vi "Get Formula String Dialog.vi"(8 "error in (no error)":errorcluster, 10 "Variable (x)":string="x", 11 "Formula Name (f(x))":string="f(x)") -> (0 "error out":errorcluster, 1 "Cancelled?":bool, 3 "Formula":string)   [LabVIEW 2019, in "XY Graph Add-Ons.lvlib"]
doc: "Displays a standard dialog box that prompts users to enter information, such as a user name and password.\n--------------------\n\nThis Express VI is configured as follows:\n\nMessage to Display to the User:\nThe inputs are: \nText Entry Box: Formula"
uses:
  XY Graph Add-Ons.lvlib
panel:
  in  "Formula":string caption="y' ="
  out "String":string="Enter formula using x as variable (e.g.: 3.0*x**2 - 4.32):"
  in  "Cancel":bool
  in  "OK":bool caption="OK2"
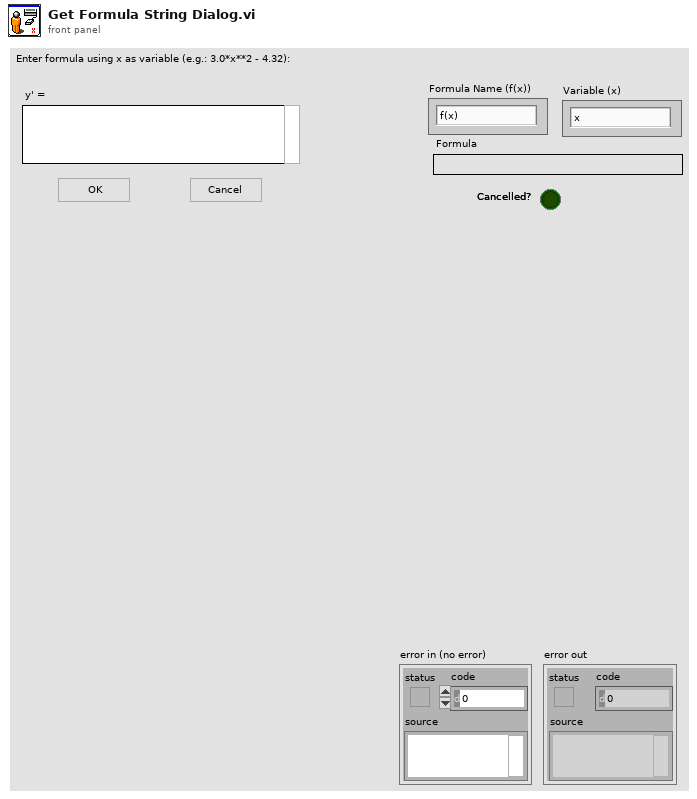
[diagram p1: front panel]
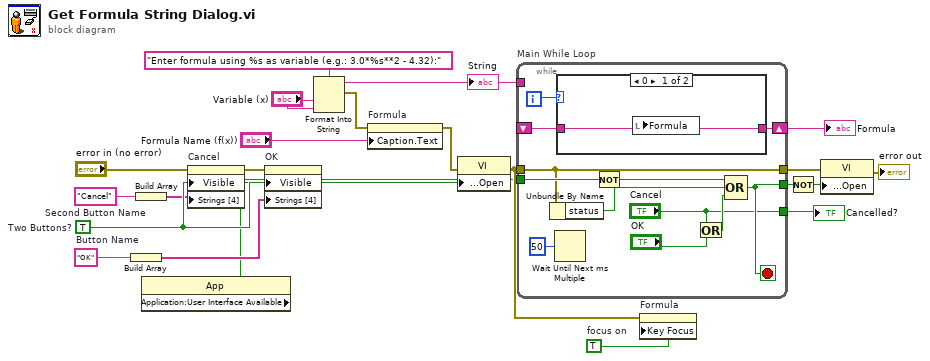
[diagram p0: block diagram]
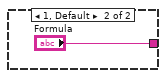
[diagram p2: hidden frame]
diagram:
  w10 = TRUE  # focus on
  w17 = "Cancel"  # Second Button Name
  w15 = "OK"  # Button Name
  w22 = TRUE  # Two Buttons?
  n1 = Build Array(w15) -> (w16:string[])
  n2 = Build Array(w17) -> (w18:string[])
  n3 = property class="App"() -> ("Application:User Interface Available"=w9:bool)  [unwired: 2 in, 2 out]
  n4 = property on="Cancel" class="Bool"(error in="error in (no error)", "Visible"=w22, "Strings [4]"=w18) -> (error out=w21:errorcluster)  [unwired: 1 in, 1 out]
  n5 = property on="OK" class="Bool"(error in=w21, "Visible"=w22, "Strings [4]"=w16) -> ()  [unwired: 1 in, 2 out]
  n6 = Format Into String(format string="Enter formula using %s as variable (e.g.: 3.0*%s**2 - 4.32):" ("Message to Display"), "Variable (x)", "Variable (x)") -> (resulting string=w6:string, error out=w2:errorcluster)  [unwired: 2 in]
  "String" <- w6
  n7 = property on="Formula" class="Str"(error in=w2, "Caption.Text"="Formula Name (f(x))") -> (error out=w3:errorcluster)  [unwired: 1 in, 1 out]
  n8 = property class="VI"(error in=w3, "Front Panel Window:Open"=w9) -> (error out=w14:errorcluster)  [unwired: 1 in, 1 out]
  n9 = while "Main While Loop" {
    tunnel: w9 -> [w33]
    tunnel: [w31] -> w19
    tunnel: w14 -> [w30]
    tunnel: [w30] -> w12
    tunnel: ["Cancel"] -> w8
    shift-right: [w24] -> w7
    shift-left: _ -> [w23]
    tunnel: w6 -> [_]
    i -> [w25]
    stop <- w31 stop-if-true
    n10 = Unbundle By Name(w30) -> ("status"=w28:bool)
    n11 = Wait Until Next ms Multiple(millisecond multiple=u32 50) -> ()  [unwired: 1 out]
    n12 = case shown="0" w25 {
      tunnel: [w35 "Formula"] -> w24
      tunnel: w23 -> [w35 _]
      frame 0 {
        n13 = local write "Formula"(w35) -> ()
      }
      frame 1, Default {
      }
    }
    n14 = Not(x=w33) -> (.not. x?=w32:bool)
    n15 = Or(x="Cancel", y="OK") -> (x .or. y?=w29:bool)
    n16 = Compound Arithmetic op=OR(w32, w28, w29) -> (w31:bool)
  }
  "Cancelled?" <- w8
  "Formula" <- w7
  n17 = property on="Formula" class="Str"(error in=w14, "Key Focus"=w10) -> ()  [unwired: 1 in, 2 out]
  n18 = Not(x=w19) -> (.not. x?=w20:bool)
  n19 = property class="VI"(error in=w12, "Front Panel Window:Open"=w20) -> (error out=→"error out":errorcluster)  [unwired: 1 in, 1 out]
